vi "current-x-pixel.vi"(7 "micrometers/pix":sgl, 10 "x(k)":sgl, 11 "xpix-n":i16) -> (2 "in-current-pix":bool, 3 "xpix(k+1)":i16)   [LabVIEW 2015]
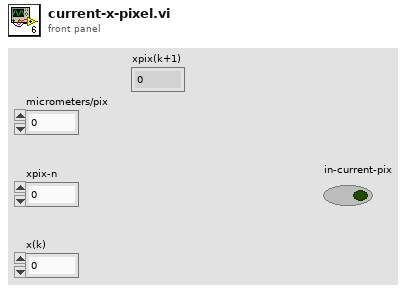
[diagram p1: front panel]
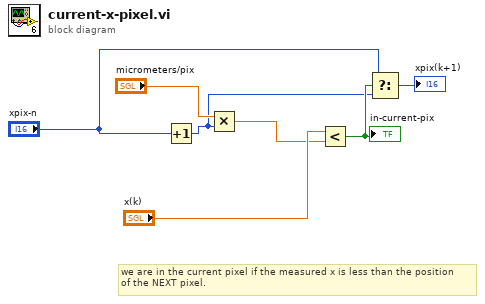
[diagram p0: block diagram]
diagram:
  # "we are in the current pixel if the measured x is less than the position\nof the NEXT pixel."
  n1 = Increment(x="xpix-n") -> (x+1=w4:i16)
  n2 = Multiply(x="micrometers/pix", y=w4) -> (x*y=w1:sgl)
  n3 = Less?(x="x(k)", y=w1) -> (x < y?=w6:bool)
  "in-current-pix" <- w6
  n4 = Select(t="xpix-n", s=w6, f=w4) -> (s? t:f=→"xpix(k+1)":i16)
